vi "Login user.vi"() -> (2 "Liste Niveau":u16, 3 "User Non Valider":bool)   [LabVIEW 2020]
uses:
  Commun VI/Library Commun.lvlib
panel:
  in  "Config Validate":bool caption="Validate"
  in  "Config Annuler":bool caption="Cancel"
  in  "MDP":string caption="Password"
  out "User":string
  in  "Liste code op":u16(ring) caption="Code User"
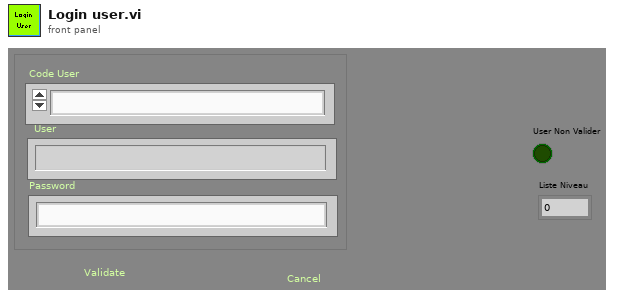
[diagram p1: front panel]
types:
  T1 = enum16{"Get Variable", "Get All Variables", "Set Variable", "Delete Variable", "Delete All Variable"}
  T2 = enum16{"Lecture Liste User", "Lecture User", "Suppression User", "Write User"}
  T3 = cluster{"Code User":string, "MDP":string, "User":string, "Liste Niveau":u16}
  T4 = enum32{"Invalid", "Standard", "Closed", "Hidden", "Minimized", "Maximized"}
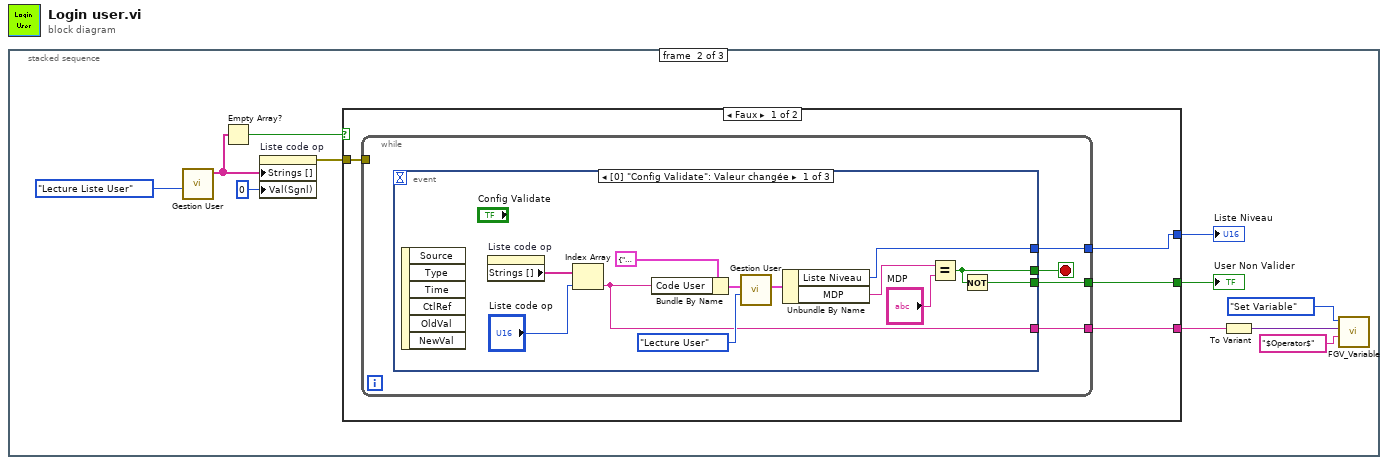
[diagram p0: block diagram]
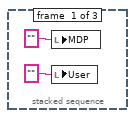
[diagram p2: hidden frame]
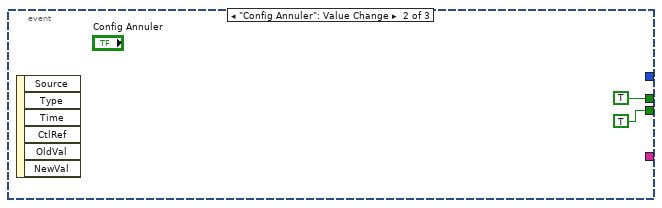
[diagram p3: hidden frame]
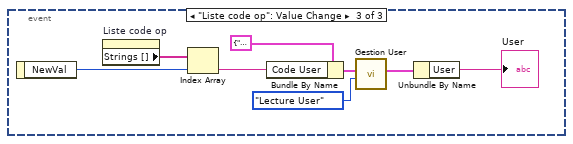
[diagram p4: hidden frame]
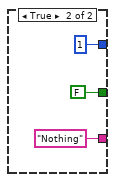
[diagram p5: hidden frame]
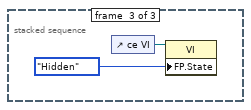
[diagram p6: hidden frame]
diagram:
  n1 = stacked-sequence {
    frame #0 {
      n2 = local write "MDP"("" ("MDP")) -> ()
      n3 = local write "User"("" ("User")) -> ()
    }
    frame #1 {
      n4 = call "Gestion User.vi"("Fonction"=T2."Lecture Liste User") -> ("Liste code Operator"=w9:string[])  [unwired: 8 in, 2 out]
      n5 = Empty Array?(array=w9) -> (empty?=w8:bool)
      n6 = property on="Liste code op" class="MDér (strict)"("Strings []"=w9, "Val(Sgnl)"=0) -> (error out=w12:errorcluster)  [unwired: 2 in, 1 out]
      n7 = case shown="Faux" w8 {
        tunnel: w12 -> [w17 _]
        tunnel: [w16 FALSE] -> w7
        tunnel: [w15 u16 1 ("Liste Niveau")] -> w10
        tunnel: [w14 "Nothing"] -> w6
        frame False {
          n8 = while {
            tunnel: w17 -> [_]
            tunnel: [w20] -> w16
            tunnel: [w19] -> w15
            tunnel: [w18] -> w14
            stop <- w21 stop-if-true
            n9 = event shown="[0] \"Config Validate\": Valeur changée" {
              selector: _ -> [_ _ _]
              dyn-events: _ -> [_ _ _]
              timeout: _ -> [_ _ _]
              tunnel: [w25 TRUE _] -> w21
              tunnel: [w24 TRUE ("User Valider") _] -> w20
              tunnel: [w23 _ _] -> w19
              tunnel: [w22 _ _] -> w18
              event "Config Validate": Value Change {
                n10 = event-data() -> ()  [unwired: 1 in, 6 out]
                n11 = property on="Liste code op" class="MDér (strict)"() -> ("Strings []"=w31:string[])  [unwired: 2 in, 2 out]
                n12 = Index Array(array=w31, index="Liste code op") -> (element=w22:string)
                n13 = Bundle By Name(cluster=T3 {"Code User"="", "MDP"="", "User"="", "Liste Niveau"=0} ("Commade User"), "Code User"=w22) -> (w29:T3)
                n14 = call "Gestion User.vi"("Fonction"=T2."Lecture User", "Commade User"=w29) -> ("Retour User"=w28:T3)  [unwired: 7 in, 2 out]
                n15 = Unbundle By Name(w28) -> ("Liste Niveau"=w23:u16, "MDP"=w27:string)
                n16 = Equal?(x=w27, y="MDP") -> (x = y?=w25:bool)
                n17 = Not(x=w25) -> (.not. x?=w24:bool)
              }
              event "Config Annuler": Value Change {
                n18 = event-data() -> ()  [unwired: 1 in, 6 out]
              }
              event "Liste code op": Value Change {
                n19 = event-data() -> ("NewVal"=w37:u16)  [unwired: 1 in]
                n20 = property on="Liste code op" class="MDér (strict)"() -> ("Strings []"=w43:string[])  [unwired: 2 in, 2 out]
                n21 = Index Array(array=w43, index=w37) -> (element=w42:string)
                n22 = Bundle By Name(cluster=T3 {"Code User"="", "MDP"="", "User"="", "Liste Niveau"=0} ("Commade User"), "Code User"=w42) -> (w40:T3)
                n23 = call "Gestion User.vi"("Fonction"=T2."Lecture User", "Commade User"=w40) -> ("Retour User"=w38:T3)  [unwired: 7 in, 2 out]
                n24 = Unbundle By Name(w38) -> ("User"=→"User":string)
              }
            }
          }
        }
        frame True {
        }
      }
      "Liste Niveau" <- w10
      "User Non Valider" <- w7
      n25 = To Variant(anything=w6) -> (Variant=w5:variant)
      n26 = call "FGV_Variable.vi"("Variable"="$Operator$" ("Name"), "Data In"=w5, "Function"=T1."Set Variable") -> ()  [unwired: 6 in, 3 out]
    }
    frame #2 {
      n27 = control-ref of="ce VI"() -> (w48:refnum<vi>)
      n28 = property class="VI"(reference=w48, "FP.State"=T4."Hidden" ("Fenêtre face-avant:État")) -> ()  [unwired: 1 in, 2 out]
    }
  }
